vi "loadFTSUM.vi"(9 "End Date":string="2014/9/24", 11 "From Date":string="2014/9/20") -> (0 "error out":errorcluster)   [LabVIEW 2012]
uses:
  <vilib>/addons/database/Auxilliary.llb/DB Tools Cursor Type.ctl
  <vilib>/addons/database/Connection.llb/DB Tools Open Connec (Path).vi
  <vilib>/addons/database/Connection.llb/Conn Execute.vi
  <vilib>/addons/database/Recordset.llb/Rec Fetch Recordset Data (R).vi
  <vilib>/addons/database/Recordset.llb/Rec Destroy - Connection.vi
  <vilib>/addons/database/_DB Variant To Data/Database Variant To Data.xnode
  <vilib>/addons/database/NI_Database_API.lvlib
panel:
  in  "Cluster":T1
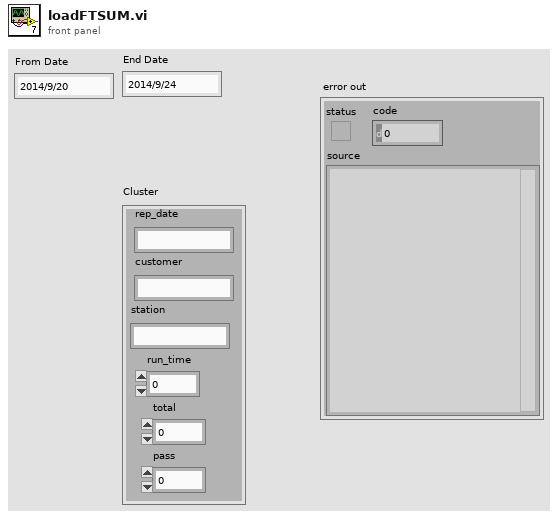
[diagram p1: front panel]
types:
  T1 = cluster{"rep_date":string, "customer":string, "station":string, "run_time":dbl, "total":dbl, "pass":dbl}
  T2 = typedef "NI_Database_API.lvlib/DB Tools Cursor Type.ctl" = enum16{"forward-only", "keyset", "dynamic", "static"}
  T3 = typedef "NI_Database_API.lvlib/Conn ObjectReference.ctl" = refnum<k1>
  T4 = typedef "NI_Database_API.lvlib/Rec ObjectReference.ctl" = refnum<k1>
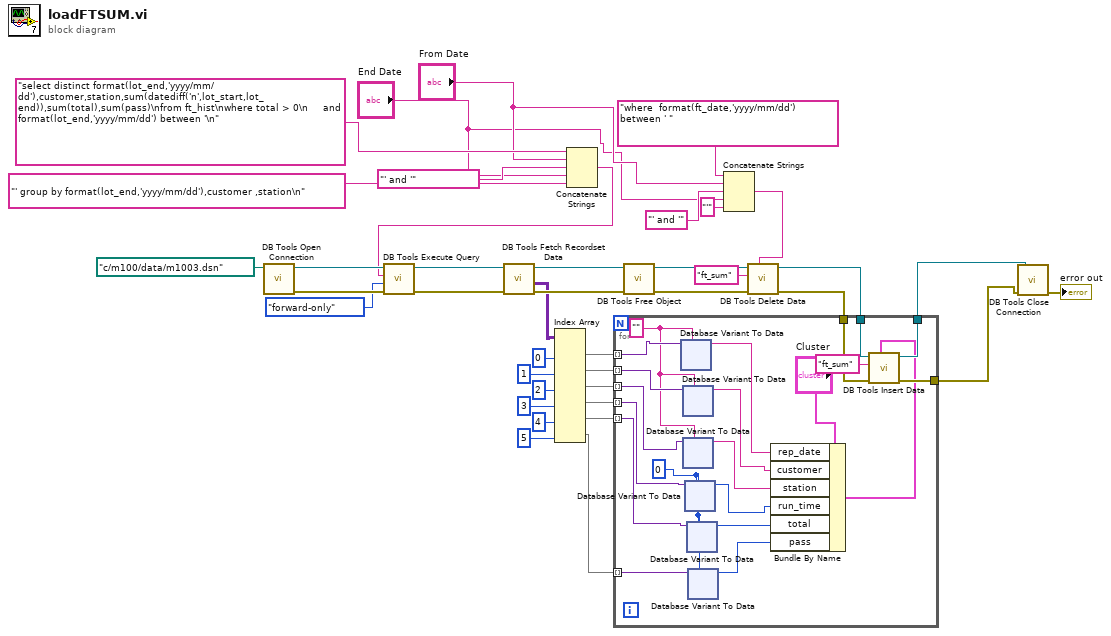
[diagram p0: block diagram]
diagram:
  n1 = call-poly <vilib>:"DB Tools Open Connection.vi"("connection information"=path "c:/m100/data/m1003.dsn") -> ("error out"=w36:errorcluster, "connection reference"=w39:T3)  [unwired: 7 in]
  n2 = Concatenate Strings("select distinct format(lot_end,'yyyy/mm/dd'),customer,station,sum(datediff('n',lot_start,lot_end)),sum(total),sum(pass)\nfrom ft_hist\nwhere total > 0\n     and  format(lot_end,'yyyy/mm/dd') between '\n" ("SQL query"), "From Date", "' and '" ("string"), "End Date", "' group by format(lot_end,'yyyy/mm/dd'),customer ,station\n" ("string")) -> (w12:string)
  n3 = call-poly <vilib>:"DB Tools Execute Query.vi"("error in (no error)"=w36, "cursor type"=DB_Tools_Cursor_Type."forward-only", "SQL query"=w12, "connection reference"=w39) -> ("error out"=w35:errorcluster, "recordset reference"=w38:T4)  [unwired: 4 in]
  n4 = call-poly <vilib>:"DB Tools Fetch Recordset Data.vi"("error in (no error)"=w35, "recordset reference"=w38) -> ("error out"=w34:errorcluster, "recordset data"=w31:variant[][], "recordset reference out"=w37:T4)  [unwired: 3 in]
  n5 = Index Array(array=w31, index (col) #1=0 ("disabled index (col)"), index (col) #2=1 ("index (col)"), index (col) #3=2 ("index (col)"), index (col) #4=3 ("index (col)"), index (col) #5=4 ("index (col)"), index (col) #6=5 ("index (col)")) -> (element #1=w27:variant[], element #2=w26:variant[], element #3=w25:variant[], element #4=w21:variant[], element #5=w20:variant[], element #6=w18:variant[])  [unwired: 6 in]
  n6 = call-poly <vilib>:"DB Tools Free Object.vi"("error in (no error)"=w34, "recordset reference"=w37) -> ("error out"=w10:errorcluster, "connection reference"=w11:T3)  [unwired: 8 in]
  n7 = Concatenate Strings("where  format(ft_date,'yyyy/mm/dd') between ' " ("string"), "From Date", "' and '" ("string"), "End Date", "'" ("string")) -> (w1:string)
  n8 = call <vilib>:"DB Tools Delete Data.vi"("condition"=w1, "error in (no error)"=w10, "table"="ft_sum", "connection reference"=w11) -> ("error out"=w9:errorcluster, "connection reference out"=w8:T3)  [unwired: 6 in]
  n9 = for {
    tunnel: w27 -> [w60] mode=indexing
    tunnel: w26 -> [w59] mode=indexing
    tunnel: w25 -> [w58] mode=indexing
    tunnel: w21 -> [w57] mode=indexing
    tunnel: w20 -> [w56] mode=indexing
    tunnel: w18 -> [w54] mode=indexing
    tunnel: w8 -> [w45]
    tunnel: w9 -> [w44]
    tunnel: [w43] -> w17
    tunnel: [w42] -> w16
    w53 = 0
    w55 = ""
    n10 = xnode "Database Variant To Data"("database variant"=w60, "type"=w55) -> ("data"=w51:string)  [unwired: 1 in, 1 out]
    n11 = xnode "Database Variant To Data"("database variant"=w59, "type"=w55) -> ("data"=w50:string)  [unwired: 1 in, 1 out]
    n12 = xnode "Database Variant To Data"("database variant"=w58, "type"=w55) -> ("data"=w49:string)  [unwired: 1 in, 1 out]
    n13 = xnode "Database Variant To Data"("database variant"=w57, "type"=w53) -> ("data"=w48:i32)  [unwired: 1 in, 1 out]
    n14 = xnode "Database Variant To Data"("database variant"=w56, "type"=w53) -> ("data"=w47:i32)  [unwired: 1 in, 1 out]
    n15 = xnode "Database Variant To Data"("database variant"=w54, "type"=w53) -> ("data"=w46:i32)  [unwired: 1 in, 1 out]
    n16 = Bundle By Name(cluster="Cluster", "rep_date"=w51, "customer"=w50, "station"=w49, "run_time"=w48, "total"=w47, "pass"=w46) -> (w41:T1)
    n17 = call <vilib>:"DB Tools Insert Data.vi"("data"=w41, "error in (no error)"=w44, "table"="ft_sum", "connection reference"=w45) -> ("error out"=w42:errorcluster, "connection reference out"=w43:T3)  [unwired: 6 in]
  }
  n18 = call <vilib>:"DB Tools Close Connection.vi"("error in (no error)"=w16, "connection reference"=w17) -> ("error out"=→"error out":errorcluster)  [unwired: 5 in]
